vi "Task Stop.vi"(8 "error in (no error)":errorcluster, 11 "LoggingManager in":refnum<class "LoggingManager.lvclass">) -> (0 "error out":errorcluster, 3 "LoggingManager out":refnum<class "LoggingManager.lvclass">)   [LabVIEW 2020, in "VolatusDataLogger.lvlib" / "LoggingManager.lvclass"]
uses:
  LoggingManager.lvclass
  LoggingManager.lvclass/LoggingManager.ctl
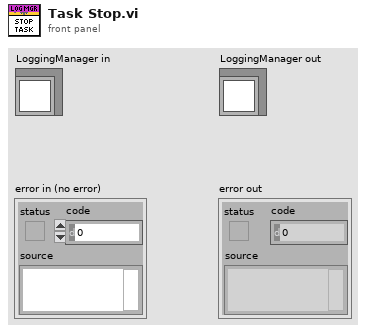
[diagram p1: front panel]
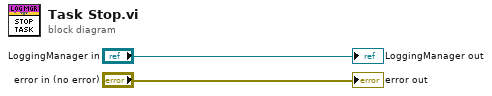
[diagram p0: block diagram]
diagram:
  "error out" <- "error in (no error)"
  "LoggingManager out" <- "LoggingManager in"
